vi "Test Xeryon API.vi"() -> ()   [LabVIEW 2019, in "Inst.Xeryon-Rotator.lvclass"]
uses:
  Inst.Xeryon-Rotator.lvclass
panel:
  out "error out":errorcluster
  out "Status":string
  out "Angle (°)":dbl
  in  "VISA resource name":refnum<visa-resource-name>
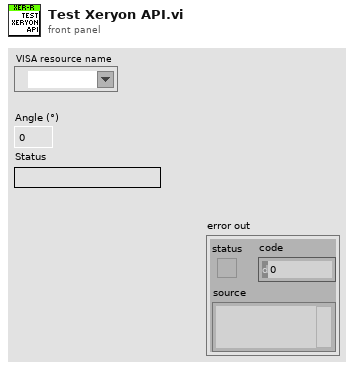
[diagram p1: front panel]
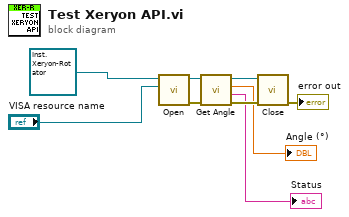
[diagram p0: block diagram]
diagram:
  n1 = call-dynamic "Open.vi"("address"="VISA resource name", "Inst.Xeryon-Rotator in"=refnum<class "Inst.Xeryon-Rotator.lvclass"> refnum) -> ("error out"=w7:errorcluster, "Inst.Xeryon-Rotator out"=w9:refnum<class "Inst.Xeryon-Rotator.lvclass">)  [unwired: 8 in]
  n2 = call-dynamic "Get Angle.vi"("error in (no error)"=w7, "Inst.Xeryon-Rotator in"=w9) -> ("error out"=w6:errorcluster, "Status"=→"Status":string, "Angle (°)"=→"Angle (°)":dbl, "Inst.Xeryon-Rotator out"=w8:refnum<class "Inst.Xeryon-Rotator.lvclass">)  [unwired: 6 in]
  n3 = call-dynamic "Close.vi"("error in (no error)"=w6, "Inst.Xeryon-Rotator in"=w8) -> ("error out"=→"error out":errorcluster)  [unwired: 8 in, 1 out]
